vi "ConfigureDlg.vi"(8 "error in (no error)":errorcluster, 11 "PmuBase in":refnum<class "Sim_Ideal_PMU.lvclass">) -> (0 "error out":errorcluster, 2 "Changed":bool, 3 "PmuBase out":refnum<class "Sim_Ideal_PMU.lvclass">)   [LabVIEW 2018, in "SensorPlugins.lvlib" / "Sim_Ideal_PMU.lvclass"]
uses:
  Sim_Ideal_PMU.lvclass
  X:/Projects/PMUCal/Modules/Sensor/SensorPlugins/PmuBaseClass/PmuBase.lvclass
  C:/Program Files (x86)/National Instruments/LabVIEW 2018/user.lib/NIST/BaseClasses/BasePlugin_class/BasePlugin.lvclass
  PmuBaseClass/Typedef/PmuConfig.ctl
  PmuBaseClass/Typedef/ePhases.ctl
  PmuBaseClass/PmuBase.lvclass/PmuBase.ctl
  Sim_Ideal_PMU.lvclass/Sim_Ideal_PMU.ctl
  <userlib>/NIST/BaseClasses/BasePlugin_class/BasePlugin.lvclass/BasePlugin.ctl
  FGen/MemberClasses/FunctionBaseClass/FunctionBase.lvclass
  PmuBaseClass/Accessors/Read PhaseArray.vi
  PmuBaseClass/Accessors/Read PmuConfig.vi
  Accessors/Read FunctionIniFilePath.vi
  <userlib>/NIST/BaseClasses/BasePlugin_class/Accessors/Read PluginIniFilePath.vi
  PmuBaseClass/Accessors/Write PmuConfig.vi
  PmuBaseClass/Accessors/Write PhaseArray.vi
  <userlib>/NIST/BaseClasses/BasePlugin_class/Accessors/Write PluginIniFilePath.vi
  Accessors/Write Function.vi
  Accessors/Write FunctionIniFilePath.vi
  Accessors/Read Function.vi
  <vilib>/Utility/error.llb/Error Cluster From Error Code.vi
  <vilib>/ErrorRing/Error Ring.xnode
  <vilib>/Utility/config.llb/NI_LVConfig.lvlib
  <userlib>/NIST/BaseClasses/Object_class/BaseObject.lvclass
  PmuBaseClass/PmuBase.lvclass
panel:
  in  "PhaseArray":T1[](array[typedef])=[enum."VA", enum."VB", enum."VC", enum."V+", enum."IA", enum."IB", enum."IC", enum."I+"]
  in  "PmuConfig":T2={"Class"=enum."M", "Fs"=60, "F0"=60, "FSamp"=60, "SettlingTime"=0.0, "T0"=0.0}
  in  "btnSaveAs":bool
  in  "btnFuncConfig":bool
  in  "BtnCancel":bool
  in  "btnSave":bool
  in  "FunctionIniFilePath":path caption="Test Function .ini File"
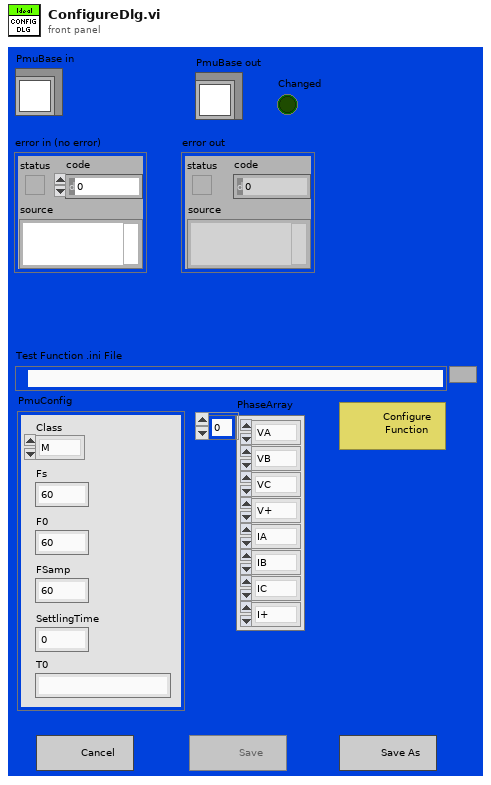
[diagram p1: front panel]
types:
  T1 = typedef "SensorPlugins.lvlib/PmuBase.lvclass/ePhases.ctl" = enum16{"VA", "VB", "VC", "V+", "IA", "IB", "IC", "I+", "none"}
  T2 = typedef "SensorPlugins.lvlib/PmuBase.lvclass/PmuConfig.ctl" = cluster{"Class":enum16{"M", "P"}, "Fs":i32, "F0":i32, "FSamp":i32, "SettlingTime":dbl, "T0":ext}
  T3 = enum32{"Invalid", "Standard", "Closed", "Hidden", "Minimized", "Maximized"}
  T4 = enum32{"Invalid", "Default", "Floating", "Floating/Auto-Hide", "Modal"}
  T5 = enum8{"Enabled", "Disabled", "Disabled and Grayed Out"}
  T6 = typedef "NI_LVConfig.lvlib/Config Data RefNum.ctl" = refnum<k1>
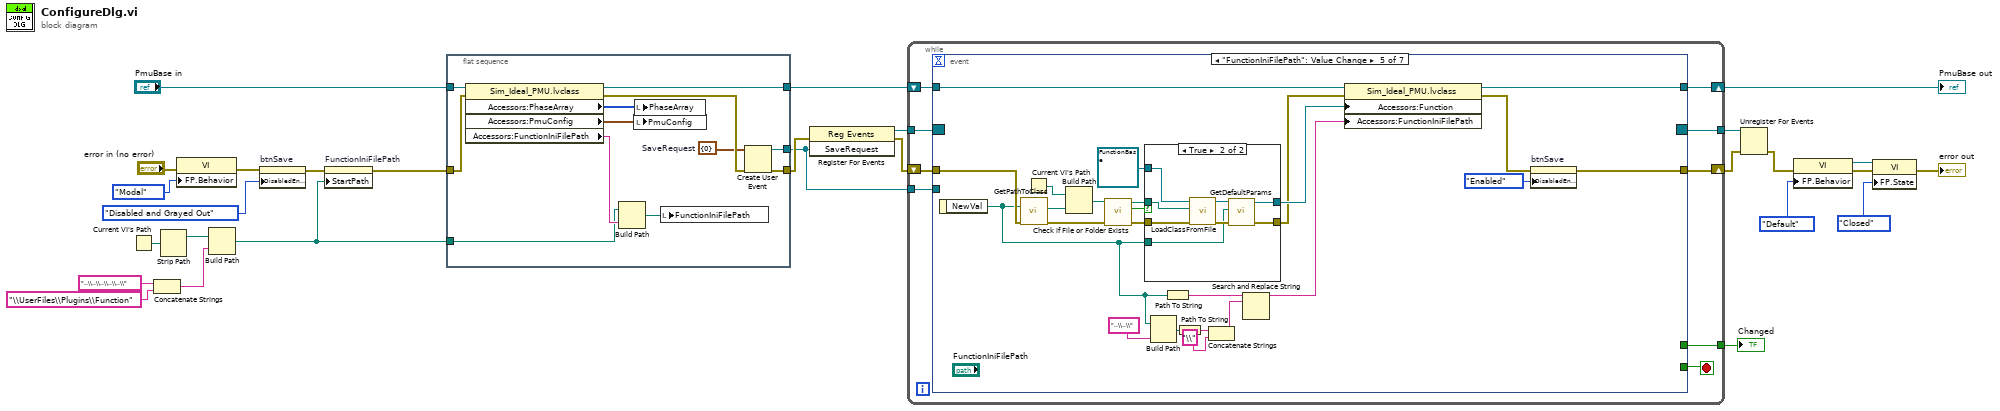
[diagram p0: block diagram]
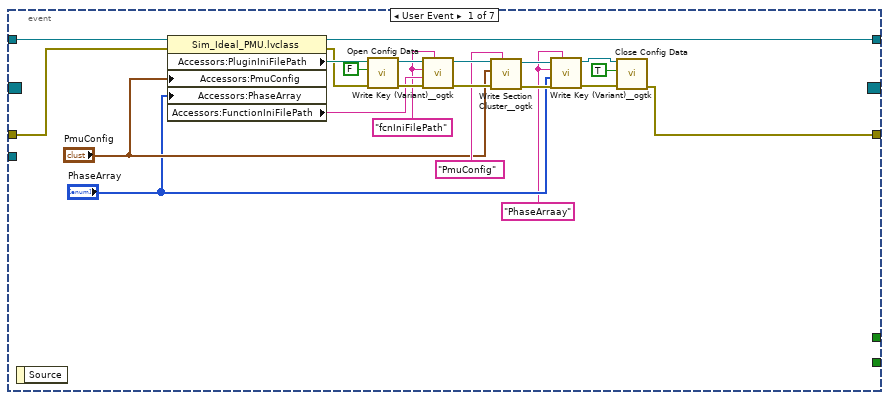
[diagram p2: hidden frame]
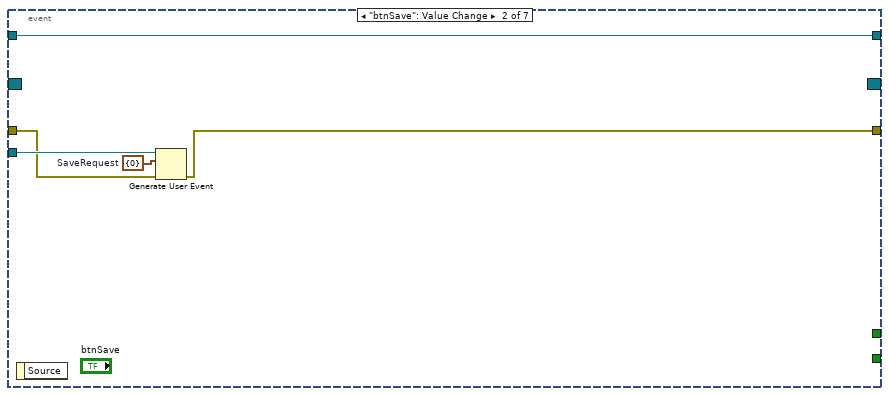
[diagram p3: hidden frame]
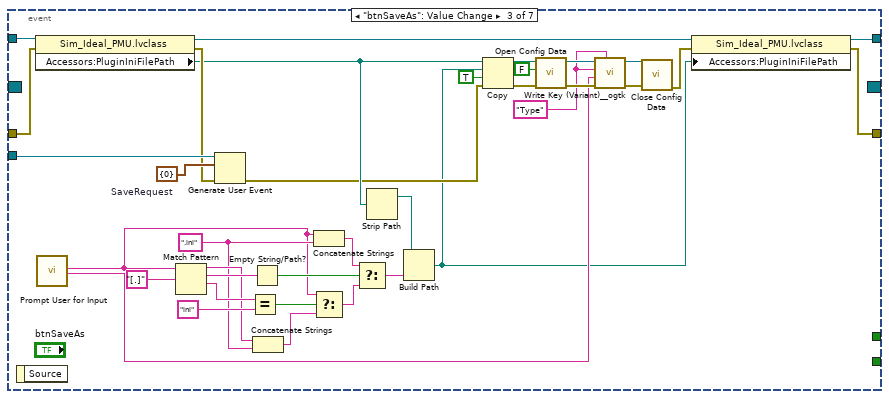
[diagram p4: hidden frame]
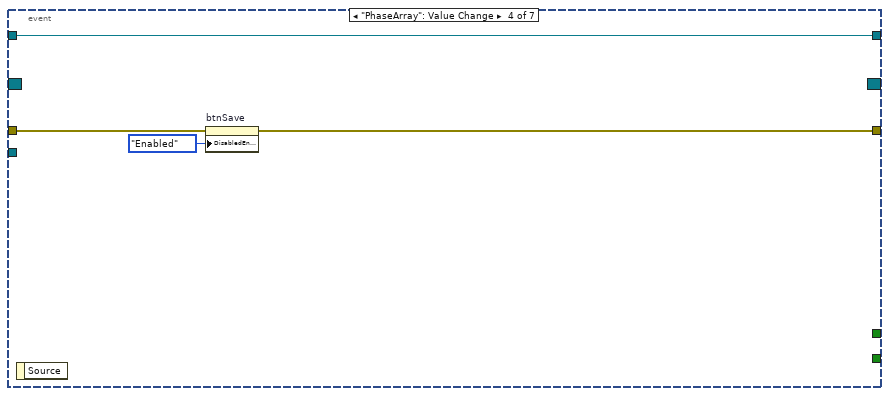
[diagram p5: hidden frame]
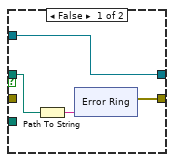
[diagram p6: hidden frame]
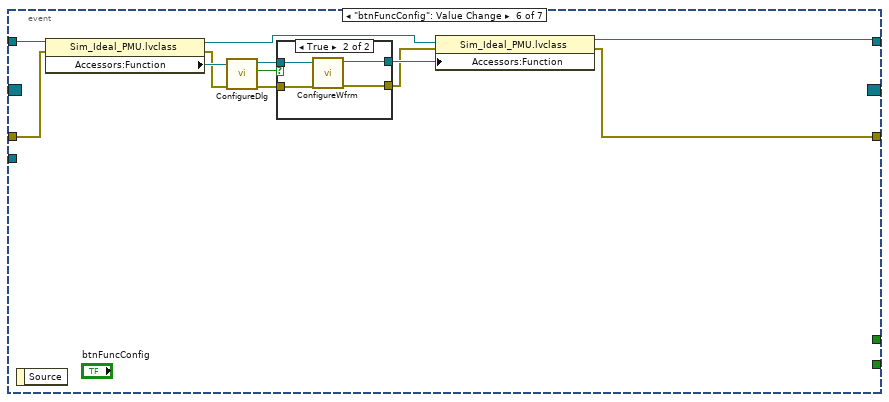
[diagram p7: hidden frame]
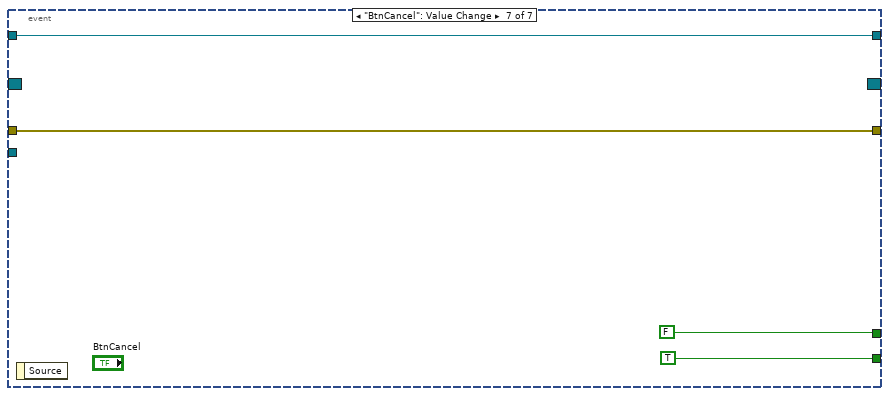
[diagram p9: hidden frame]
diagram:
  n1 = Current VI's Path() -> (path=w25:path)
  n2 = Concatenate Strings("..\\..\\..\\..\\..\\", "\\UserFiles\\Plugins\\Function" ("name or relative path")) -> (w23:string)
  n3 = Strip Path(path=w25) -> (stripped path=w22:path)  [unwired: 1 out]
  n4 = property class="VI"(error in="error in (no error)", "FP.Behavior"=T4."Modal" ("Front Panel Window:Behavior")) -> (error out=w13:errorcluster)  [unwired: 1 in, 1 out]
  n5 = Build Path(base path=w22, name or relative path=w23) -> (appended path=w10:path)
  n6 = property on="btnSave" class="Bool"(error in=w13, "DisabledEnum"=T5."Disabled and Grayed Out" ("Disabled")) -> (error out=w15:errorcluster)  [unwired: 1 in, 1 out]
  n7 = property on="FunctionIniFilePath" class="Path"(error in=w15, "StartPath"=w10) -> (error out=w11:errorcluster)  [unwired: 1 in, 1 out]
  n8 = flat-sequence {
    tunnel: "PmuBase in" -> [w40]
    tunnel: [w39] -> w12
    tunnel: w11 -> [w38]
    tunnel: [w31] -> w3
    tunnel: w10 -> [w34]
    tunnel: [w29] -> w2
    frame #0 {
      w30 = cluster{"Num":i32} {"Num"=0}  # SaveRequest
      n9 = property class="Sim_Ideal_PMU.lvclass"(reference=w40, error in=w38) -> (reference out=w39:refnum<class "Sim_Ideal_PMU.lvclass">, error out=w32:errorcluster, "Accessors:PhaseArray"=w37:T1[], "Accessors:PmuConfig"=w36:T2, "Accessors:FunctionIniFilePath"=w35:string)
      n10 = Build Path(base path=w34, name or relative path=w35) -> (appended path=w33:path)
      n11 = local write "PmuConfig"(w36) -> ()
      n12 = local write "PhaseArray"(w37) -> ()
      n13 = local write "FunctionIniFilePath"(w33) -> ()
      n14 = Create User Event(user event datatype=w30, error in=w32) -> (user event=w29:refnum<user-event>, error out=w31:errorcluster)
    }
  }
  n15 = register-events(error in=w3, w2) -> (reference out=w8:refnum<event-registration>, error out=w7:errorcluster)  [unwired: 1 in]
  n16 = while {
    shift-right: [w48] -> w9
    shift-left: w12 -> [w49]
    shift-right: [w46] -> w6
    shift-left: w7 -> [w47]
    tunnel: w8 -> [w45]
    tunnel: [w44] -> w5
    tunnel: w2 -> [w43]
    tunnel: [w41] -> w1
    stop <- w42 stop-if-true
    n17 = event shown="[4] \"FunctionIniFilePath\": Value Change" {
      selector: w45 -> [_ _ _ _ _ _ _]
      dyn-events: [_ _ _ _ _ _ _] -> w44
      timeout: _ -> [_ _ _ _ _ _ _]
      tunnel: w49 -> [w71 w76 w100 w116 w124 w171 w179]
      tunnel: [w70 w76 w80 w116 w117 w161 w179] -> w48
      tunnel: w47 -> [w69 w73 w99 w115 w140 w170 w178]
      tunnel: [w59 w72 w78 w113 w119 w160 w178] -> w46
      tunnel: w43 -> [_ w75 w98 _ _ _ _]
      tunnel: [_ _ _ _ _ _ TRUE] -> w42
      tunnel: [_ _ _ _ _ _ FALSE] -> w41
      event User Event {
        w55 = "fcnIniFilePath" ("section (optional)")
        w52 = "PhaseArraay" ("section")
        n18 = event-data() -> ()  [unwired: 1 in, 1 out]
        n19 = property class="Sim_Ideal_PMU.lvclass"(reference=w71, error in=w69, "Accessors:PmuConfig"="PmuConfig", "Accessors:PhaseArray"="PhaseArray") -> (reference out=w70:refnum<class "Sim_Ideal_PMU.lvclass">, error out=w66:errorcluster, "Accessors:PluginIniFilePath"=w68:path, "Accessors:FunctionIniFilePath"=w56:string)
        n20 = call <vilib>:"Open Config Data.vi"("error in (no error)"=w66, "create file if necessary (T)"=FALSE, "configuration file path"=w68) -> ("error out"=w65:errorcluster, "refnum"=w64:T6)  [unwired: 6 in, 1 out]
        n21 = call <userlib>:"Write Key (Variant)__ogtk.vi"("section"=w55, "error in (no error)"=w65, "key-value"=w56, "key (optional)"=w55, "refnum"=w64) -> ("error out"=w63:errorcluster, "refnum out"=w62:T6)  [unwired: 5 in]
        n22 = call <userlib>:"Write Section Cluster__ogtk.vi"("section (optional)"="PmuConfig", "error in (no error)"=w63, "Section Formatted Cluster"="PmuConfig", "refnum"=w62) -> ("error out"=w58:errorcluster, "dup refnum"=w57:T6)  [unwired: 6 in]
        n23 = call <userlib>:"Write Key (Variant)__ogtk.vi"("section"=w52, "error in (no error)"=w58, "key-value"="PhaseArray", "key (optional)"=w52, "refnum"=w57) -> ("error out"=w51:errorcluster, "refnum out"=w50:T6)  [unwired: 5 in]
        n24 = call <vilib>:"Close Config Data.vi"("error in (no error)"=w51, "write file if changed (T)"=TRUE, "refnum"=w50) -> ("error out"=w59:errorcluster)  [unwired: 7 in, 1 out]
      }
      event "btnSave": Value Change {
        w74 = cluster{"Num":i32} {"Num"=0}  # SaveRequest
        n25 = event-data() -> ()  [unwired: 1 in, 1 out]
        n26 = Generate User Event(user event=w75, event data cluster=w74, error in=w73) -> (error out=w72:errorcluster)  [unwired: 1 in, 1 out]
      }
      event "btnSaveAs": Value Change {
        w85 = "Type"
        w97 = cluster{"Num":i32} {"Num"=0}  # SaveRequest
        w105 = ".ini" ("string")
        n27 = event-data() -> ()  [unwired: 1 in, 1 out]
        n28 = property class="Sim_Ideal_PMU.lvclass"(reference=w100, error in=w99) -> (reference out=w86:refnum<class "Sim_Ideal_PMU.lvclass">, error out=w96:errorcluster, "Accessors:PluginIniFilePath"=w94:path)
        n29 = call "Prompt User for Input"() -> ("File Name"=w82:string, "PluginType Name"=w81:string)  [unwired: 16 in, 2 out]
        n30 = Match Pattern(string=w82, regular expression="[.]" ("string")) -> (before substring=w108:string, match substring=w110:string, after substring=w111:string)  [unwired: 1 in, 1 out]
        n31 = Generate User Event(user event=w98, event data cluster=w97, error in=w96) -> (error out=w92:errorcluster)  [unwired: 1 in, 1 out]
        n32 = Equal?(x=w111, y="ini" ("string")) -> (x = y?=w107:bool)
        n33 = Empty String/Path?(string/path=w110) -> (empty?=w104:bool)
        n34 = Concatenate Strings(w108, w105) -> (w106:string)
        n35 = Concatenate Strings(w82, w105) -> (w102:string)
        n36 = Select(t=w82, s=w107, f=w106) -> (s? t:f=w103:string)
        n37 = Select(t=w102, s=w104, f=w103) -> (s? t:f=w101:string)
        n38 = Strip Path(path=w94) -> (stripped path=w95:path)  [unwired: 1 out]
        n39 = Build Path(base path=w95, name or relative path=w101) -> (appended path=w77:path)
        n40 = Copy(8:w92, 9:TRUE ("overwrite (F)"), 10:w77, 11:w94) -> (0:w91:errorcluster, 3:w90:path)  [unwired: 1 in, 1 out]
        n41 = call <vilib>:"Open Config Data.vi"("error in (no error)"=w91, "create file if necessary (T)"=FALSE, "configuration file path"=w90) -> ("error out"=w88:errorcluster, "refnum"=w87:T6)  [unwired: 6 in, 1 out]
        n42 = call <userlib>:"Write Key (Variant)__ogtk.vi"("section"=w85, "error in (no error)"=w88, "key-value"=w81, "key (optional)"=w85, "refnum"=w87) -> ("error out"=w84:errorcluster, "refnum out"=w83:T6)  [unwired: 5 in]
        n43 = call <vilib>:"Close Config Data.vi"("error in (no error)"=w84, "refnum"=w83) -> ("error out"=w79:errorcluster)  [unwired: 8 in, 1 out]
        n44 = property class="Sim_Ideal_PMU.lvclass"(reference=w86, error in=w79, "Accessors:PluginIniFilePath"=w77) -> (reference out=w80:refnum<class "Sim_Ideal_PMU.lvclass">, error out=w78:errorcluster)
      }
      event "PhaseArray": Value Change {
        n45 = event-data() -> ()  [unwired: 1 in, 1 out]
        n46 = property on="btnSave" class="Bool"(error in=w115, "DisabledEnum"=T5."Enabled" ("Disabled")) -> (error out=w113:errorcluster)  [unwired: 1 in, 1 out]
      }
      event "FunctionIniFilePath": Value Change {
        n47 = event-data() -> ("NewVal"=w125:path)  [unwired: 1 in]
        n48 = call <userlib>:"GetPathToClass.vi"("error in (no error)"=w140, "configuration file path"=w125) -> ("error IO"=w136:errorcluster, "PathToClass"=w139:path)  [unwired: 8 in]
        n49 = Current VI's Path() -> (path=w138:path)
        n50 = Build Path(base path=w138, name or relative path=w139) -> (appended path=w137:path)
        n51 = call <vilib>:"Check if File or Folder Exists.vi"("error in (no error)"=w136, "path"=w137) -> ("error out"=w133:errorcluster, "file or folder exists?"=w135:bool, "dup path"=w134:path)  [unwired: 7 in]
        n52 = case shown="True" w135 {
          tunnel: w134 -> [w143 w159]
          tunnel: w133 -> [_ w157]
          tunnel: refnum<class "FunctionBase.lvclass"> refnum ("Functions.lvlib:FunctionBase.lvclass") -> [w141 w158]
          tunnel: w125 -> [_ w154]
          tunnel: [w142 w153] -> w121
          tunnel: [w141 w152] -> w123
          frame False {
            n53 = Path To String(path=w143) -> (string=w144:string)
            n54 = xnode "Error Ring"("parameter 0"=w144) -> ("error out"=w142:errorcluster)
          }
          frame True {
            n55 = call-dynamic "LoadClassFromFile.vi"("error in (no error)"=w157, "class path"=w159, "reference in"=w158) -> ("error out"=w156:errorcluster, "reference out"=w155:refnum<class "FunctionBase.lvclass">)  [unwired: 7 in]
            n56 = call-dynamic "GetDefaultParams.vi"("error in (no error)"=w156, "Path"=w154, "FunctionBase in"=w155) -> ("error out"=w153:errorcluster, "FunctionBase out"=w152:refnum<class "FunctionBase.lvclass">)  [unwired: 7 in]
          }
        }
        n57 = Build Path(base path=w125, name or relative path="..\\..\\") -> (appended path=w129:path)
        n58 = Path To String(path=w125) -> (string=w130:string)
        n59 = Path To String(path=w129) -> (string=w128:string)
        n60 = Concatenate Strings(w128, "\\" ("string")) -> (w126:string)
        n61 = Search and Replace String(input string=w130, search string=w126) -> (result string=w122:string)  [unwired: 6 in, 3 out]
        n62 = property class="Sim_Ideal_PMU.lvclass"(reference=w124, error in=w121, "Accessors:Function"=w123, "Accessors:FunctionIniFilePath"=w122) -> (reference out=w117:refnum<class "Sim_Ideal_PMU.lvclass">, error out=w120:errorcluster)
        n63 = property on="btnSave" class="Bool"(error in=w120, "DisabledEnum"=T5."Enabled" ("Disabled")) -> (error out=w119:errorcluster)  [unwired: 1 in, 1 out]
      }
      event "btnFuncConfig": Value Change {
        n64 = event-data() -> ()  [unwired: 1 in, 1 out]
        n65 = property class="Sim_Ideal_PMU.lvclass"(reference=w171, error in=w170) -> (reference out=w162:refnum<class "Sim_Ideal_PMU.lvclass">, error out=w168:errorcluster, "Accessors:Function"=w169:refnum<class "FunctionBase.lvclass">)
        n66 = call-dynamic "ConfigureDlg.vi"("error in (no error)"=w168, "FunctionBase in"=w169) -> ("error out"=w166:errorcluster, "Changed"=w167:bool, "FunctionBase out"=w165:refnum<class "FunctionBase.lvclass">)  [unwired: 7 in]
        n67 = case shown="True" w167 {
          tunnel: w166 -> [w173 w176]
          tunnel: w165 -> [w172 w177]
          tunnel: [w173 w175] -> w163
          tunnel: [w172 w174] -> w164
          frame False {
          }
          frame True {
            n68 = call-dynamic "ConfigureWfrm.vi"("error in (no error)"=w176, "FunctionBase in"=w177) -> ("error out"=w175:errorcluster, "FunctionBase out"=w174:refnum<class "FunctionBase.lvclass">)  [unwired: 8 in]
          }
        }
        n69 = property class="Sim_Ideal_PMU.lvclass"(reference=w162, error in=w163, "Accessors:Function"=w164) -> (reference out=w161:refnum<class "Sim_Ideal_PMU.lvclass">, error out=w160:errorcluster)
      }
      event "BtnCancel": Value Change {
        n70 = event-data() -> ()  [unwired: 1 in, 1 out]
      }
    }
  }
  "PmuBase out" <- w9
  "Changed" <- w1
  n71 = Unregister For Events(event registration refnum=w5, error in=w6) -> (error out=w4:errorcluster)
  n72 = property class="VI"(error in=w4, "FP.Behavior"=T4."Default" ("Front Panel Window:Behavior")) -> (reference out=w18:refnum<vi>, error out=w19:errorcluster)  [unwired: 1 in]
  n73 = property class="VI"(reference=w18, error in=w19, "FP.State"=T3."Closed" ("Front Panel Window:State")) -> (error out=→"error out":errorcluster)  [unwired: 1 out]
